vi "ev Next frame.vi"(8 "error in (no error)":errorcluster, 11 "IDE simple in":refnum<class "Main Panel.lvclass">) -> (0 "error out":errorcluster, 3 "IDE simple out":refnum<class "Main Panel.lvclass">)   [LabVIEW 2018, in "Main Panel.lvlib" / "Main Panel.lvclass"]
uses:
  Main Panel.lvclass
  Main Panel.lvclass/Main Panel.ctl
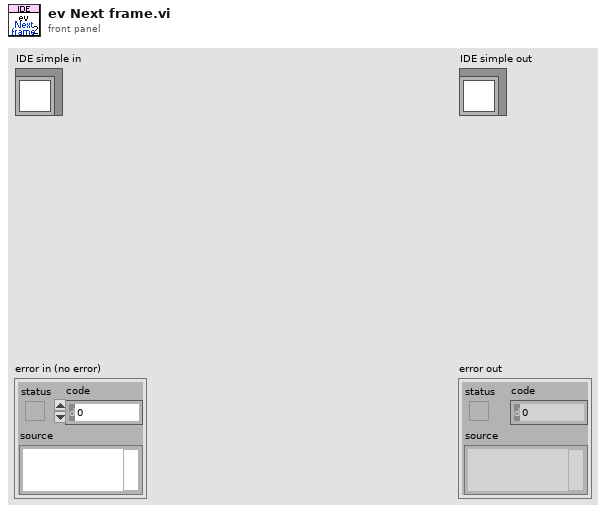
[diagram p1: front panel]
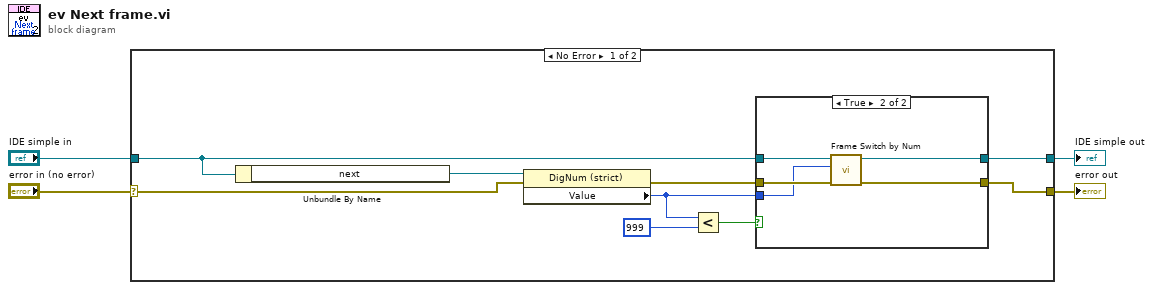
[diagram p0: block diagram]
diagram:
  n1 = case shown="No Error" "error in (no error)" {
    selector: "error in (no error)" -> [w12 w22]
    tunnel: [w9 w22] -> w3
    tunnel: [w10 w21] -> w1
    tunnel: "IDE simple in" -> [w11 w21]
    frame No Error {
      n2 = Unbundle By Name(w11) -> ("next"=w13:refnum<vi>)
      n3 = property class="DigNum (strict)"(reference=w13, error in=w12) -> (error out=w8:errorcluster, "Value"=w5:u32)  [unwired: 1 out]
      n4 = Less?(x=w5, y=u32 999) -> (x < y?=w6:bool)
      n5 = case shown="True" w6 {
        tunnel: w11 -> [w15 w20]
        tunnel: [w15 w19] -> w10
        tunnel: [w14 w18] -> w9
        tunnel: w8 -> [w14 w17]
        tunnel: w5 -> [_ w16]
        frame False {
        }
        frame True {
          n6 = call "Frame Switch by Num.vi"("error in (no error)"=w17, "Frame Num"=w16, "LF2R IDE in"=w20) -> ("error out"=w18:errorcluster, "LF2R IDE out"=w19:refnum<class "Main Panel.lvclass">)  [unwired: 7 in]
        }
      }
    }
    frame Error {
    }
  }
  "error out" <- w3
  "IDE simple out" <- w1
